vi "UserVars-Read Table.vi"(0 ".NET Refnum":refnum<k24>, 11 "error in (no error)":errorcluster) -> (8 "UserVars":T1[](array[typedef]), 15 "error out":errorcluster)   [LabVIEW 2015]
uses:
  D:/Experiment VIs/Utility VIs/User Variables/dotNET Source/UserVariableControls/bin/Release/UserVariableControls.dll
  dotNET Source/UserVariableControls/bin/Release/UserVariableControls.dll
  Tosca/LV Source/Typedefs/Tosca-Rove Variable.ctl
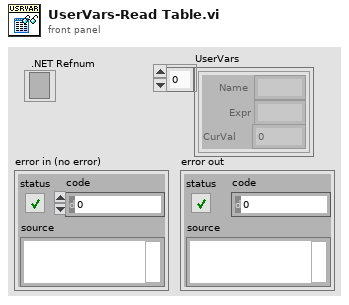
[diagram p1: front panel]
types:
  T1 = typedef "Tosca-Rove Variable.ctl" = cluster{"Name":string, "Expr":string, "CurVal":dbl}
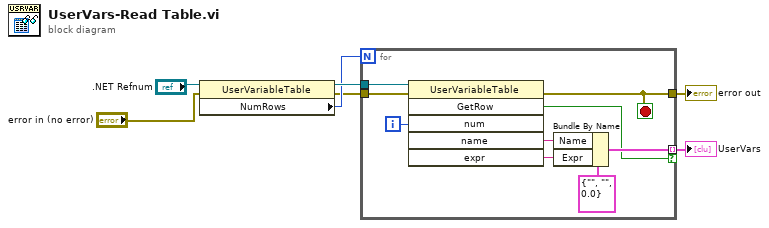
[diagram p0: block diagram]
diagram:
  n1 = property class="UserVariableTable"(reference=".NET Refnum", error in="error in (no error)") -> (reference out=w6:refnum<k24>, error out=w2:errorcluster, "NumRows"=w5:i32)
  n2 = for {
    N: w5 -> [_]
    tunnel: w6 -> [w16]
    tunnel: [w12] -> w4 mode=indexing if=w11
    tunnel: w2 -> [w9]
    tunnel: [w8] -> w1
    i -> [w10]
    stop <- w8 stop-if-true
    n3 = invoke class="UserVariableTable" method="GetRow"(reference=w16, error in=w9, "num"=w10) -> (error out=w8:errorcluster, "GetRow"=w11:bool, "name"=w14:string, "expr"=w13:string)  [unwired: 3 in, 2 out]
    n4 = Bundle By Name(cluster=T1 {"Name"="", "Expr"="", "CurVal"=0.0} ("Var"), "Name"=w14, "Expr"=w13) -> (w12:T1)
  }
  "UserVars" <- w4
  "error out" <- w1
